vi "getSize.vi"(8 "error in (no error)":errorcluster, 11 "Bucket in":refnum<class "Bucket.lvclass">) -> (0 "error out":errorcluster, 2 "Size":u32, 3 "Bucket out":refnum<class "Bucket.lvclass">)   [LabVIEW 2017, in "Bucket.lvclass"]
uses:
  <userlib>/836-Library/Data_Structures/Bucket/Bucket.lvclass
  <userlib>/836-Library/Data_Structures/Bucket/Bucket.lvclass/Bucket.ctl
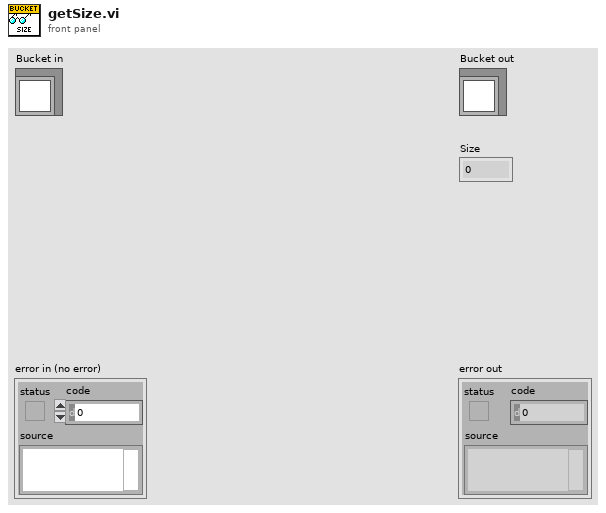
[diagram p1: front panel]
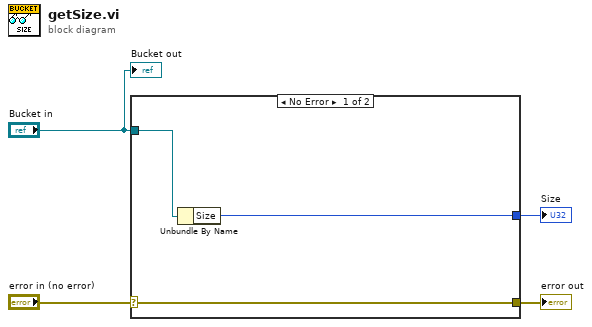
[diagram p0: block diagram]
diagram:
  n1 = case shown="No Error" "error in (no error)" {
    selector: "error in (no error)" -> [w7 w8]
    tunnel: [w7 w8] -> w3
    tunnel: "Bucket in" -> [w6 _]
    tunnel: [w5 _] -> w2
    frame No Error {
      n2 = Unbundle By Name(w6) -> ("Size"=w5:u32)
    }
    frame Error {
    }
  }
  "error out" <- w3
  "Size" <- w2
  "Bucket out" <- "Bucket in"
